vi "NT_LL_Read Boolean.vi"(8 "error in (no error)":errorcluster, 10 "default value":bool, 11 "subscribeHandle":u32) -> (0 "error out":errorcluster, 2 "time":i64, 3 "Boolean":bool)   [LabVIEW 2025]
uses:
  FRC_NetworkTablesLV.dll
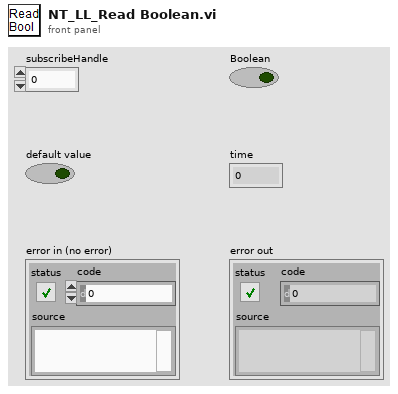
[diagram p1: front panel]
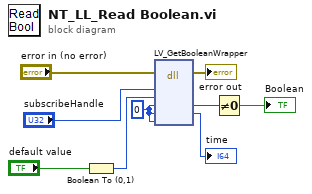
[diagram p0: block diagram]
diagram:
  w9 = 0 ("readValue")
  n1 = Boolean To (0,1)(Boolean="default value") -> (0, 1=w3:i16)
  n2 = dll-call lib="FRC_NetworkTablesLV.*" fn="LV_GetBooleanWrapper"(error in="error in (no error)", "subscribeHandle"="subscribeHandle", "default"=w3, "readValue"=w9, "time"=w9, "serverTime"=w9) -> (error out=→"error out":errorcluster, "readValue"=w6:i32, "time"=→"time":i64)  [unwired: 6 in, 1 out]
  n3 = Not Equal To 0?(x=w6) -> (x != 0?=→"Boolean":bool)
